vi "Display Serial Number Table.vi"() -> ()   [LabVIEW 2010]
uses:
  <vilib>/Utility/miscctls.llb/LVDateTimeRec.ctl
  <vilib>/Utility/miscctls.llb/LVRowAndColumnTypeDef.ctl
  <vilib>/Utility/file.llb/Read From Spreadsheet File (string).vi
  <vilib>/Utility/file.llb/Write To Spreadsheet File (string).vi
panel:
  in  "Save":bool
  in  "Exit":bool
  in  "Table Control":string[][](table)
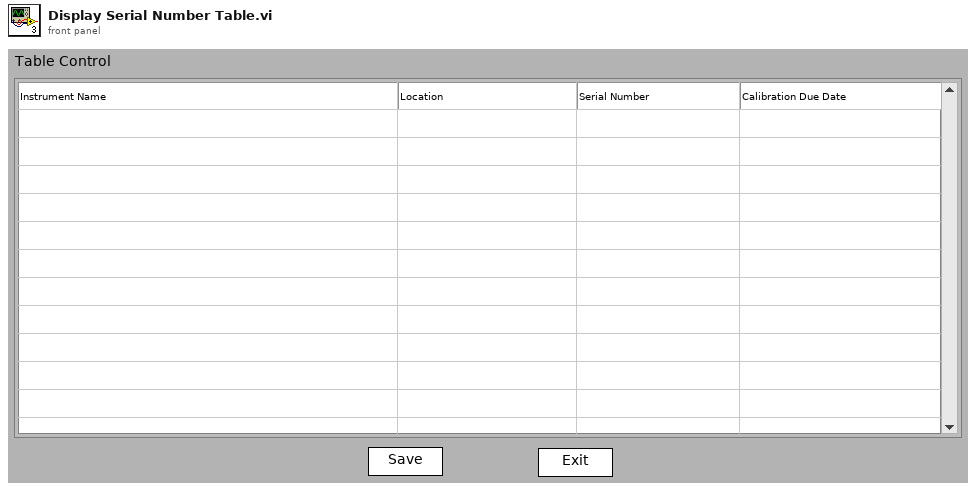
[diagram p1: front panel]
types:
  T1 = typedef "LVDateTimeRec.ctl" = cluster{"fractional second":dbl, "second":i32, "minute":i32, "hour":i32, "day of month":i32, "month":i32, "year":i32, "day of week":i32, "day of year":i32, "DST":i32}
  T2 = typedef "LVRowAndColumnTypeDef.ctl" = cluster{"Row":i32, "Column":i32}
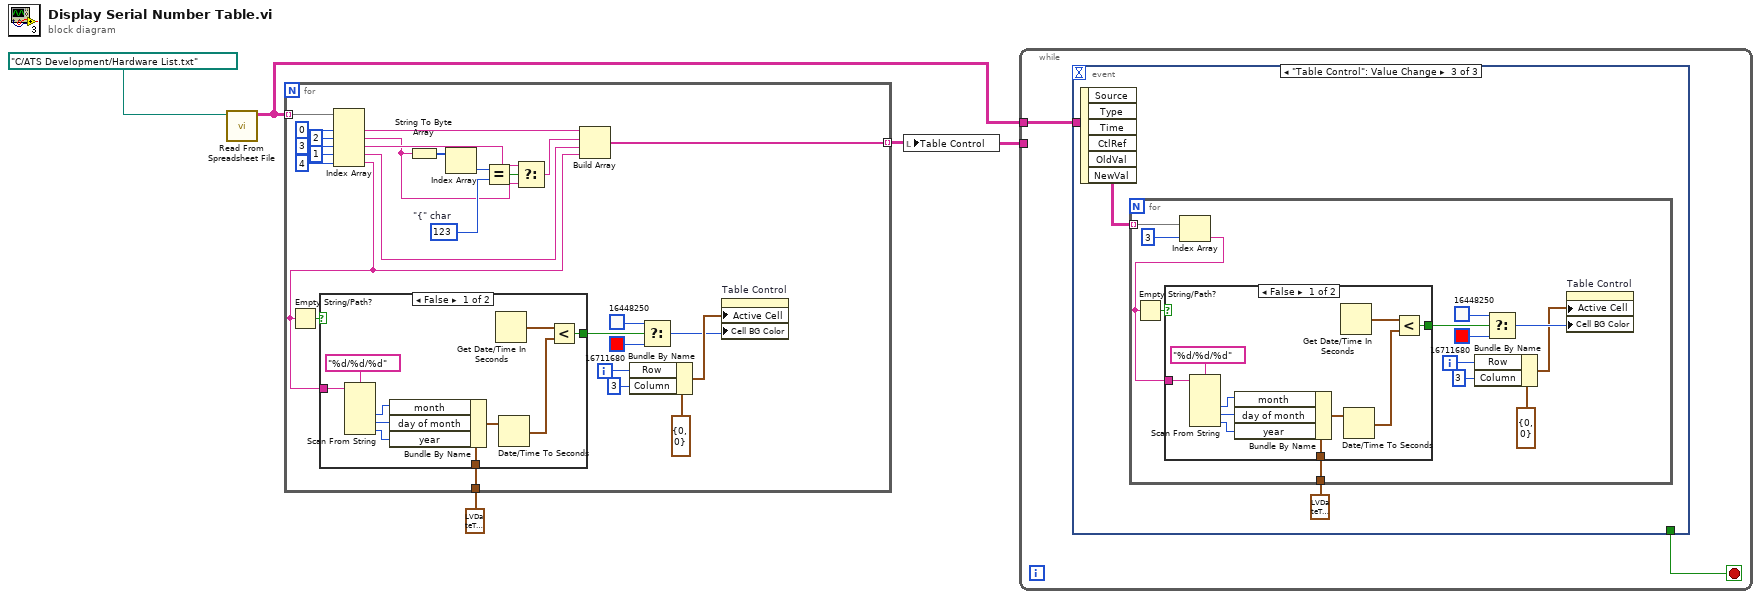
[diagram p0: block diagram]
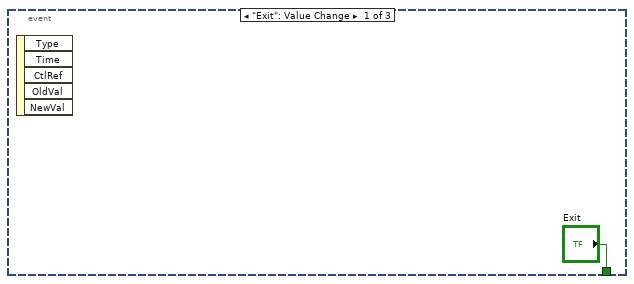
[diagram p2: hidden frame]
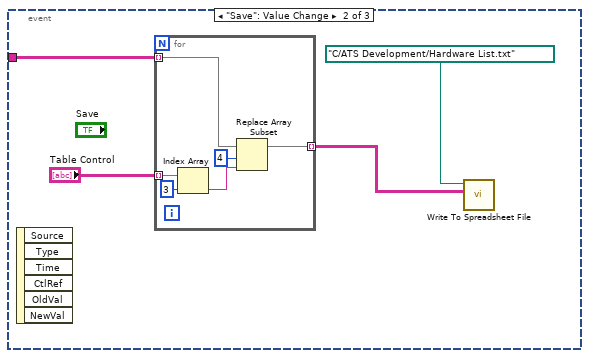
[diagram p3: hidden frame]
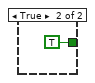
[diagram p4: hidden frame]
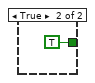
[diagram p5: hidden frame]
diagram:
  n1 = call-poly <vilib>:"Read From Spreadsheet File.vi"("file path (dialog if empty)"=path "C:/ATS Development/Hardware List.txt") -> ("all rows"=w2:string[][])  [unwired: 6 in, 4 out]
  n2 = for {
    tunnel: w2 -> [w31] mode=indexing
    tunnel: [w16] -> w3 mode=indexing
    tunnel: T1 {"fractional second"=0.0, "second"=0, "minute"=0, "hour"=0, "day of month"=0, "month"=0, "year"=0, "day of week"=0, "day of year"=0, "DST"=0} ("date time rec") -> [w8]
    i -> [w13]
    w21 = u8 123  # "{" char
    n3 = Index Array(array=w31, index #1=0 ("index"), index #2=2 ("index"), index #3=3 ("index"), index #4=1 ("index"), index #5=4 ("index")) -> (element #1=w25:string, element #2=w18:string, element #3=w19:string, element #4=w24:string, element #5=w5:string)
    n4 = Empty String/Path?(string/path=w5) -> (empty?=w6:bool)
    n5 = case shown="False" w6 {
      tunnel: w8 -> [w40 _]
      tunnel: w5 -> [w35 _]
      tunnel: [w32 TRUE] -> w7
      frame False {
        n6 = Scan From String(format string="%d/%d/%d", input string=w35) -> (output 1=w38:i32, output 2=w37:i32, output 3=w36:i32)  [unwired: 5 in, 3 out]
        n7 = Bundle By Name(cluster=w40, "month"=w38, "day of month"=w37, "year"=w36) -> (w39:T1)
        n8 = Get Date/Time In Seconds() -> (seconds since 1Jan1904=w34:timestamp)
        n9 = Date/Time To Seconds(2:w39) -> (0:w33:timestamp)  [unwired: 1 in]
        n10 = Less?(x=w34, y=w33) -> (x < y?=w32:bool)
      }
      frame True {
      }
    }
    n11 = String To Byte Array(string=w18) -> (unsigned byte array=w23:u8[])
    n12 = Index Array(array=w23) -> (element=w22:u8)  [unwired: 1 in]
    n13 = Equal?(x=w22, y=w21) -> (x = y?=w20:bool)
    n14 = Select(t=w19, s=w20, f=w18) -> (s? t:f=w17:string)
    n15 = Build Array(w25, w17, w24, w5) -> (w16:string[])
    n16 = Bundle By Name(cluster=T2 {"Row"=0, "Column"=0} ("Active Cell:Active Cell"), "Row"=w13, "Column"=3) -> (w14:T2)
    n17 = Select(t=u32 16448250, s=w7, f=u32 16711680) -> (s? t:f=w9:u32)
    n18 = property on="Table Control" class="Tbl (strict)"("Active Cell"=w14, "Cell BG Color"=w9) -> ()  [unwired: 2 in, 2 out]
  }
  n19 = local write "Table Control"(w3) -> ()
  n20 = while {
    tunnel: w3 -> [_]
    tunnel: w2 -> [w43]
    stop <- w44 stop-if-true
    n21 = event shown="[2] \"Table Control\": Value Change" {
      selector: _ -> [_ _ _]
      dyn-events: _ -> [_ _ _]
      timeout: _ -> [_ _ _]
      tunnel: ["Exit" _ _] -> w44
      tunnel: w43 -> [_ w48 _]
      event "Exit": Value Change {
        n22 = event-data() -> ()  [unwired: 1 in, 5 out]
      }
      event "Save": Value Change {
        n23 = event-data() -> ()  [unwired: 1 in, 6 out]
        n24 = for {
          tunnel: w48 -> [w53] mode=indexing
          tunnel: "Table Control" -> [w55] mode=indexing
          tunnel: [w50] -> w46 mode=indexing
          n25 = Index Array(array=w55, index=3) -> (element=w52:string)
          n26 = Replace Array Subset(array=w53, new element=w52, index=4) -> (w50:string[])
        }
        n27 = call-poly <vilib>:"Write To Spreadsheet File.vi"("2D data"=w46, "file path (dialog if empty)"=path "C:/ATS Development/Hardware List.txt") -> ()  [unwired: 6 in, 1 out]
      }
      event "Table Control": Value Change {
        n28 = event-data() -> ("NewVal"=w56:string[][])  [unwired: 1 in, 5 out]
        n29 = for {
          tunnel: T1 {"fractional second"=0.0, "second"=0, "minute"=0, "hour"=0, "day of month"=0, "month"=0, "year"=0, "day of week"=0, "day of year"=0, "DST"=0} ("date time rec") -> [w64]
          tunnel: w56 -> [w60] mode=indexing
          i -> [w68]
          n30 = Index Array(array=w60, index=3) -> (element=w61:string)
          n31 = Empty String/Path?(string/path=w61) -> (empty?=w62:bool)
          n32 = case shown="False" w62 {
            tunnel: w64 -> [w79 _]
            tunnel: w61 -> [w74 _]
            tunnel: [w71 TRUE] -> w63
            frame False {
              n33 = Scan From String(format string="%d/%d/%d", input string=w74) -> (output 1=w77:i32, output 2=w76:i32, output 3=w75:i32)  [unwired: 5 in, 3 out]
              n34 = Bundle By Name(cluster=w79, "month"=w77, "day of month"=w76, "year"=w75) -> (w78:T1)
              n35 = Get Date/Time In Seconds() -> (seconds since 1Jan1904=w73:timestamp)
              n36 = Date/Time To Seconds(2:w78) -> (0:w72:timestamp)  [unwired: 1 in]
              n37 = Less?(x=w73, y=w72) -> (x < y?=w71:bool)
            }
            frame True {
            }
          }
          n38 = Bundle By Name(cluster=T2 {"Row"=0, "Column"=0} ("Active Cell:Active Cell"), "Row"=w68, "Column"=3) -> (w58:T2)
          n39 = Select(t=u32 16448250, s=w63, f=u32 16711680) -> (s? t:f=w59:u32)
          n40 = property on="Table Control" class="Tbl (strict)"("Active Cell"=w58, "Cell BG Color"=w59) -> ()  [unwired: 2 in, 2 out]
        }
      }
    }
  }
